vi "send_stop_notification.vi"(1 "Should stop":bool, 2 "Stop notification queue":refnum<queue>) -> (0 "Queue out":refnum<queue>)   [LabVIEW 2010]
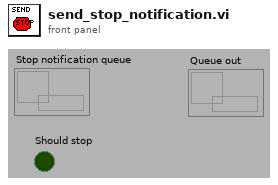
[diagram p1: front panel]
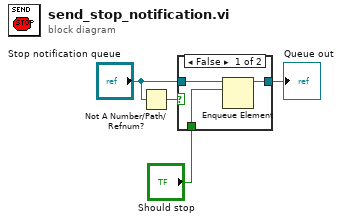
[diagram p0: block diagram]
diagram:
  n1 = Not A Number/Path/Refnum?(number/path/refnum="Stop notification queue") -> (NaN/Path/Refnum?=w3:bool)
  n2 = case shown="False" w3 {
    tunnel: "Stop notification queue" -> [w7 w8]
    tunnel: [w6 w8] -> w2
    tunnel: "Should stop" -> [w5 _]
    frame False {
      n3 = Enqueue Element(queue=w7, element=w5) -> (queue out=w6:refnum<queue>)  [unwired: 2 in, 2 out]
    }
    frame True {
    }
  }
  "Queue out" <- w2
